vi "Get Audio Spectrum Notifier.vi"(8 "Error In":errorcluster, 11 "Audio Analyzer In":refnum<class "Audio Analyzer.lvclass">) -> (0 "Error Out":errorcluster, 2 "Audio Spectrum Notifier":refnum<notifier>, 3 "Audio Analyzer Out":refnum<class "Audio Analyzer.lvclass">)   [LabVIEW 2021, in "Audio Analyzer.lvclass"]
uses:
  Audio Analyzer.lvclass
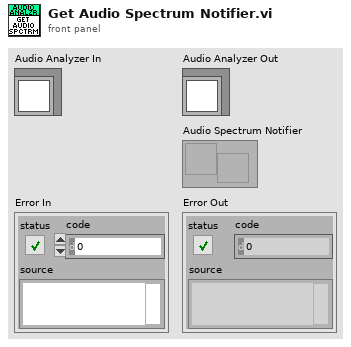
[diagram p1: front panel]
types:
  T1 = typedef "Audio Analyzer.lvclass/Data.ctl" = cluster{"Audio Spectrum Notifier":refnum<notifier>, "FPGA Reference":T2}
  T2 = typedef "Audio Analyzer.lvclass/FPGA Reference.ctl" = refnum<k20>
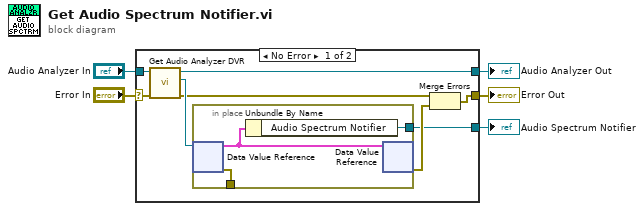
[diagram p0: block diagram]
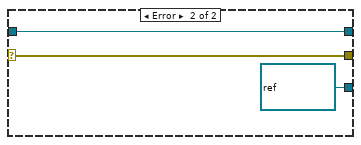
[diagram p2: hidden frame]
diagram:
  n1 = case shown="No Error" "Error In" {
    selector: "Error In" -> [w9 w18]
    tunnel: [w11 w18] -> w2
    tunnel: [w8 w19] -> w4
    tunnel: "Audio Analyzer In" -> [w10 w19]
    tunnel: [w12 refnum<notifier> refnum ("Audio Spectrum Notifier")] -> w1
    frame No Error {
      n2 = call "Get Audio Analyzer DVR.vi"("Error In"=w9, "Audio Analyzer In"=w10) -> ("Error Out"=w6:errorcluster, "DVR"=w7:refnum<data-value>, "Audio Analyzer Out"=w8:refnum<class "Audio Analyzer.lvclass">)  [unwired: 7 in]
      n3 = in-place {
        in-place-border: [w14] -> w12
        in-place-border: [w16] -> _
        n4 = in-place-dvr #1(w7) -> (w15:T1, w16:errorcluster)
        n5 = Unbundle By Name(w15) -> ("Audio Spectrum Notifier"=w14:refnum<notifier>)
        n6 = in-place-dvr #1(w15) -> (w13:errorcluster)  [unwired: 1 out]
      }
      n7 = Merge Errors(w6, w13) -> (w11:errorcluster)
    }
    frame Error {
    }
  }
  "Audio Analyzer Out" <- w4
  "Error Out" <- w2
  "Audio Spectrum Notifier" <- w1
